vi "Temperture Warnings.vi"() -> ()   [LabVIEW 2015]
doc: "Wejścia: Temparatura aktualna, maksymalna oraz minimalna\nWyjscia: Ostrzezenie LED oraz tekst ostrzeżenia\nAdrianna Graja \n05.11.2017"
panel:
  out "Warning text":string
  out "Warning?":bool
  in  "Min Temperature":dbl
  in  "Max Temperature":dbl
  in  "Current Temperature":dbl
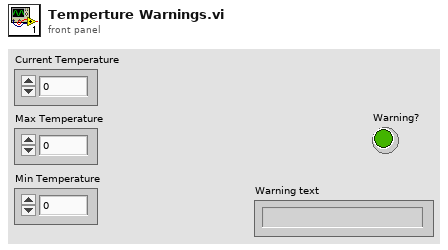
[diagram p1: front panel]
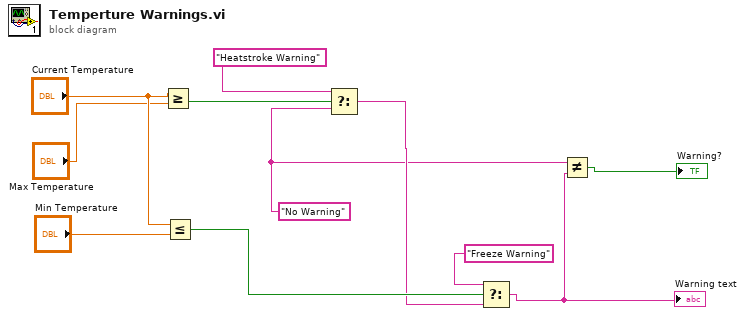
[diagram p0: block diagram]
diagram:
  w3 = "No Warning"
  n1 = Greater Or Equal?(x="Current Temperature", y="Max Temperature") -> (x >= y?=w11:bool)
  n2 = Less Or Equal?(x="Current Temperature", y="Min Temperature") -> (x <= y?=w9:bool)
  n3 = Select(t="Heatstroke Warning", s=w11, f=w3) -> (s? t:f=w8:string)
  n4 = Select(t="Freeze Warning", s=w9, f=w8) -> (s? t:f=w1:string)
  "Warning text" <- w1
  n5 = Not Equal?(x=w3, y=w1) -> (x != y?=→"Warning?":bool)
